vi "Think.vi"(1 "Enum":enum16{"Running", "Impact", "Spinning", "Clear"}(ring)) -> (0 "Enum 2":enum16{"Running", "Impact", "Spinning", "Clear"}(ring))   [LabVIEW 2010]
uses:
  Main Global.vi
panel:
  out "Radius":dbl
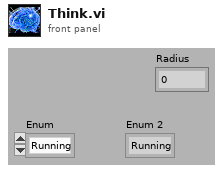
[diagram p1: front panel]
types:
  T1 = typedef "Streaming Data.ctl" = cluster{"Bump Right":bool, "Bump Left":bool, "Wheel Drop Right":bool, "Wheel Drop Left":bool, "Wheel Drop Caster":bool, "Wall":bool, "Cliff Left":bool, "Cliff Front Left":bool, "Cliff Front Right":bool, "Cliff Right":bool, "IR Red":bool, "IR Green":bool, "IR Force":bool, "Play":bool, "Advance":bool, "Battery Charge":i16}
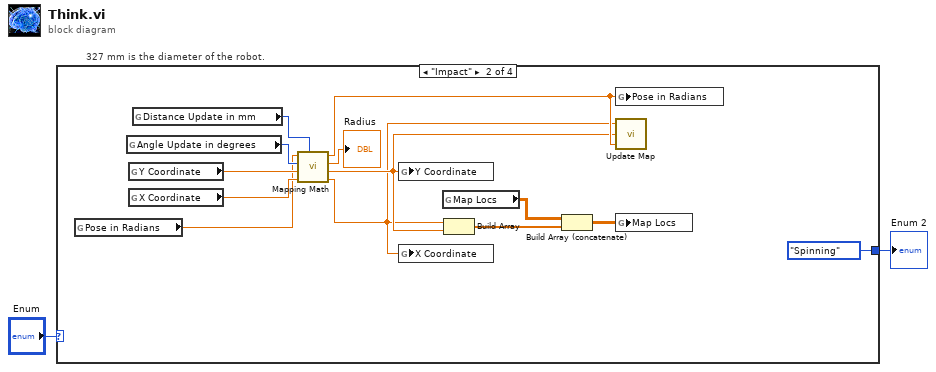
[diagram p0: block diagram]
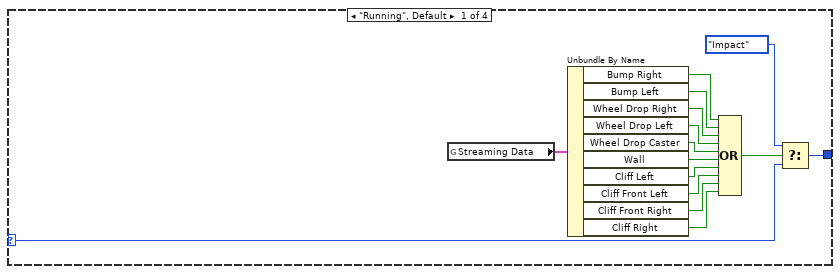
[diagram p2: hidden frame]
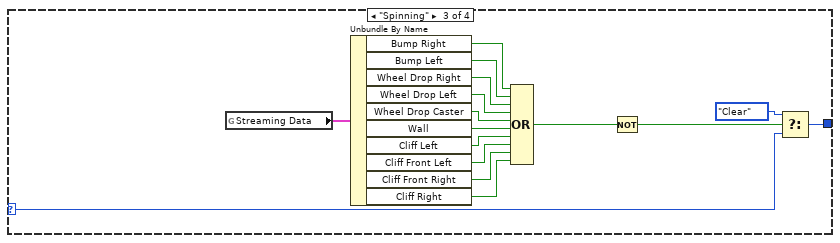
[diagram p3: hidden frame]
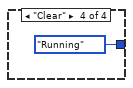
[diagram p4: hidden frame]
diagram:
  # "327 mm is the diameter of the robot."
  n1 = case shown="\"Impact\"" "Enum" {
    selector: "Enum" -> [w17 _ w33 _]
    tunnel: [w16 enum16{"Running", "Impact", "Spinning", "Clear"}."Spinning" w31 enum16{"Running", "Impact", "Spinning", "Clear"}."Running" ("t")] -> w1
    frame "Running", Default {
      n2 = global read "Main Global.vi" "Streaming Data"() -> (w15:T1)
      n3 = Unbundle By Name(w15) -> ("Bump Right"=w14:bool, "Bump Left"=w13:bool, "Wheel Drop Right"=w12:bool, "Wheel Drop Left"=w11:bool, "Wheel Drop Caster"=w10:bool, "Wall"=w9:bool, "Cliff Left"=w8:bool, "Cliff Front Left"=w7:bool, "Cliff Front Right"=w6:bool, "Cliff Right"=w5:bool)
      n4 = Compound Arithmetic op=OR(w14, w13, w12, w11, w10, w9, w8, w7, w6, w5) -> (w4:bool)
      n5 = Select(t=enum16{"Running", "Impact", "Spinning", "Clear"}."Impact", s=w4, f=w17) -> (s? t:f=w16:enum16{"Running", "Impact", "Spinning", "Clear"})
    }
    frame "Impact" {
      n6 = global read "Main Global.vi" "Pose in Radians"() -> (w21:dbl)
      n7 = global read "Main Global.vi" "Angle Update in degrees"() -> (w30:i16)
      n8 = global read "Main Global.vi" "Y Coordinate"() -> (w22:dbl)
      n9 = global read "Main Global.vi" "X Coordinate"() -> (w23:dbl)
      n10 = global read "Main Global.vi" "Distance Update in mm"() -> (w29:i16)
      n11 = call "Mapping Math.vi"("Distance Update in mm"=w29, "X Coordinate"=w23, "Y Coordinate"=w22, "Angle Update in degrees"=w30, "Pose in Radians"=w21) -> ("X out"=w18:dbl, "Y out"=w19:dbl, "Radius"=→"Radius":dbl, "Pose Out"=w20:dbl)
      n12 = global write "Main Global.vi" "Y Coordinate"(w19) -> ()
      n13 = global write "Main Global.vi" "X Coordinate"(w18) -> ()
      n14 = global read "Main Global.vi" "Map Locs"() -> (w26:dbl[][])
      n15 = Build Array(w18, w19) -> (w27:dbl[])
      n16 = Build Array (concatenate)(w26, w27) -> (w25:dbl[][])
      n17 = global write "Main Global.vi" "Pose in Radians"(w20) -> ()
      n18 = call "Update Map.vi"("Pose in Radians"=w20, "Y"=w19, "X"=w18) -> ()
      n19 = global write "Main Global.vi" "Map Locs"(w25) -> ()
    }
    frame "Spinning" {
      n20 = global read "Main Global.vi" "Streaming Data"() -> (w46:T1)
      n21 = Unbundle By Name(w46) -> ("Bump Right"=w45:bool, "Bump Left"=w44:bool, "Wheel Drop Right"=w43:bool, "Wheel Drop Left"=w42:bool, "Wheel Drop Caster"=w41:bool, "Wall"=w40:bool, "Cliff Left"=w39:bool, "Cliff Front Left"=w38:bool, "Cliff Front Right"=w37:bool, "Cliff Right"=w36:bool)
      n22 = Compound Arithmetic op=OR(w45, w44, w43, w42, w41, w40, w39, w38, w37, w36) -> (w35:bool)
      n23 = Not(x=w35) -> (.not. x?=w34:bool)
      n24 = Select(t=enum16{"Running", "Impact", "Spinning", "Clear"}."Clear", s=w34, f=w33) -> (s? t:f=w31:enum16{"Running", "Impact", "Spinning", "Clear"})
    }
    frame "Clear" {
    }
  }
  "Enum 2" <- w1
